vi "NavX Subsystem.vi"   [LabVIEW 2016]
uses:
  <vilib>/Rock Robotics/SystemInterfaces/i2clib/i2c_bus.ctl
  NavX Global.vi
  <vilib>/Rock Robotics/Network Tables/NT Write Number.vi
  <vilib>/Rock Robotics/WPI/ThirdParty/Sensors/navX/_Processing Loop/FRIC_navX_Internal_I2C_ProcessingLoop.vi
types:
  T1 = typedef "i2c_bus.ctl" = enum16{"I2C On-Board", "I2C MXP", "Invalid"}
  T2 = cluster{"Yaw":dbl, "Roll":dbl, "Pitch":dbl, "Heading":dbl, "Fused Heading":dbl}
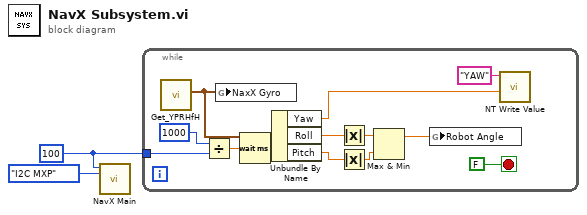
[diagram p0: block diagram]
diagram:
  w1 = u8 100 ("Rate (4Hz-200Hz)")
  n1 = call-poly <vilib>:"NavX Main.vi"("I2C Bus"=i2c_bus."I2C MXP", "Rate (4Hz-200Hz)"=w1) -> ()  [unwired: 10 in]
  n2 = while {
    tunnel: w1 -> [w12]
    stop <- FALSE stop-if-true
    n3 = call <vilib>:"Get_YPRHfH.vi"() -> ("YRPHfH"=w9:T2)  [unwired: 11 in]
    n4 = Divide(x=1000, y=w12) -> (x/y=w11:dbl)
    n5 = global write "NavX Global.vi" "NaxX Gyro"(w9) -> ()
    n6 = Wait (ms)(milliseconds to wait=w11) -> ()  [unwired: 1 out]
    n7 = Unbundle By Name(w9) -> ("Yaw"=w8:dbl, "Roll"=w6:dbl, "Pitch"=w7:dbl)
    n8 = Absolute Value(x=w6) -> (abs(x)=w5:dbl)
    n9 = Absolute Value(x=w7) -> (abs(x)=w4:dbl)
    n10 = Max & Min(x=w5, y=w4) -> (max(x,y)=w3:dbl)  [unwired: 1 out]
    n11 = global write "NavX Global.vi" "Robot Angle"(w3) -> ()
    n12 = call-poly <vilib>:"NT Write Value.vi"("Numeric"=w8, "Name"="YAW") -> ()  [unwired: 9 in, 1 out]
  }
